vi "WFS Error-Query.vi"(8 "error in (no error)":errorcluster {"code" format="%.0x"}, 11 "instrument handle":refnum<visa-resource-name>) -> (0 "error out":errorcluster {"code" format="%.0x"}, 1 "Error Message":string, 2 "Error Code":i32 format="%.0g", 3 "instrument handle out":refnum<visa-resource-name>)   [LabVIEW 2020]
doc: "This VI queries the instrument and returns instrument-specific error information."
uses:
  WFS_32.dll
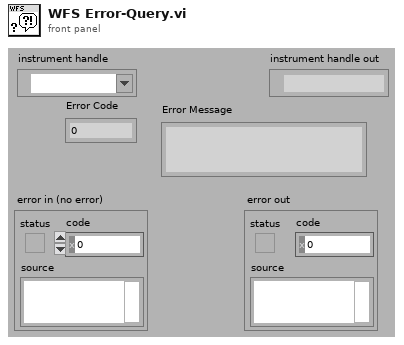
[diagram p1: front panel]
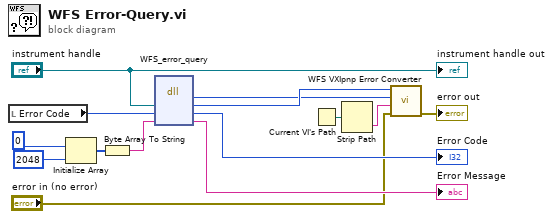
[diagram p0: block diagram]
diagram:
  n1 = local read "Error Code"() -> (w11:i32)
  n2 = Initialize Array(u8 0, 2048 ("size of error message")) -> (w12:u8[])
  n3 = Byte Array To String(unsigned byte array=w12) -> (string=w9:string)
  n4 = dll-call lib="WFS_*.*" fn="WFS_error_query"("instrument handle"="instrument handle", "error code"=w11, "error message"=w9) -> ("Status"=w4:i32, "instrument handle"=w5:u32, "error code"=→"Error Code":i32, "error message"=→"Error Message":string)  [unwired: 3 in, 2 out]
  n5 = Current VI's Path() -> (path=w7:path)
  n6 = Strip Path(path=w7) -> (name=w3:string)  [unwired: 1 out]
  n7 = call "WFS VXIpnp Error Converter.vi"("error in (no error)"="error in (no error)", "Name Of VI (\"\")"=w3, "CVI Error Code (0)"=w4, "instrument handle"=w5) -> ("error out"=→"error out":errorcluster)  [unwired: 6 in, 1 out]
  "instrument handle out" <- "instrument handle"
